vi "CleanUp.vi"(0 "object in":refnum<class "Hamamatsu.lvclass">, 5 "error in (no error)":errorcluster) -> (14 "object out":refnum<class "Hamamatsu.lvclass">, 19 "error out":errorcluster)   [LabVIEW 2021, in "Hamamatsu.lvclass"]
uses:
  Hamamatsu.lvclass
  Hamamatsu.lvclass/Hamamatsu.ctl
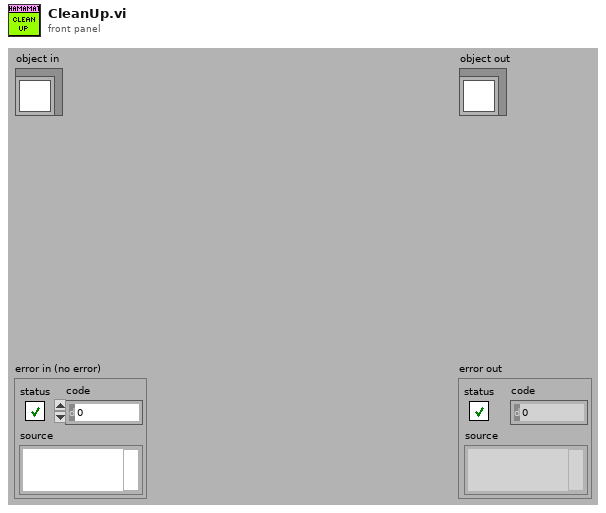
[diagram p1: front panel]
types:
  T1 = typedef "IMAQ Image.ctl" = refnum<image>
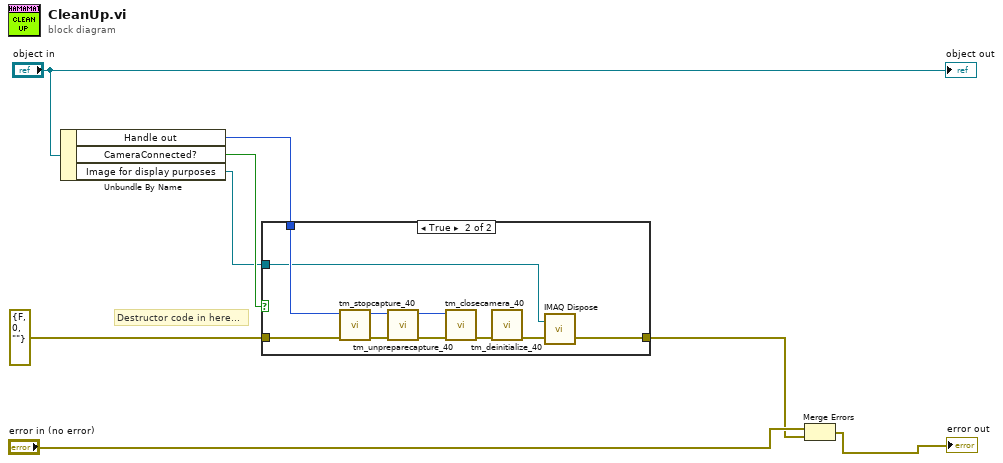
[diagram p0: block diagram]
diagram:
  # "Destructor code in here..."
  n1 = Unbundle By Name("object in") -> ("Handle out"=w5:u32, "CameraConnected?"=w2:bool, "Image for display purposes"=w1:T1)
  n2 = case shown="True" w2 {
    tunnel: w5 -> [_ w13]
    tunnel: errorcluster {"status"=FALSE, "code"=0, "source"=""} ("error in (no error)") -> [w9 w15]
    tunnel: [w9 w10] -> w3
    tunnel: w1 -> [_ w12]
    frame False {
    }
    frame True {
      n3 = call <userlib>:"tm_stopcapture_40.vi"("error in (no error)"=w15, "Handle in"=w13) -> ("error out"=w17:errorcluster, "Handle out"=w18:u32)  [unwired: 8 in]
      n4 = call <userlib>:"tm_unpreparecapture_40.vi"("error in (no error)"=w17, "Handle in"=w18) -> ("error out"=w16:errorcluster, "Handle out"=w14:u32)  [unwired: 8 in]
      n5 = call <userlib>:"tm_closecamera_40.vi"("error in (no error)"=w16, "Handle in"=w14) -> ("error out"=w19:errorcluster)  [unwired: 9 in]
      n6 = call <userlib>:"tm_deinitialize_40.vi"("error in (no error)"=w19) -> ("error out"=w11:errorcluster)  [unwired: 10 in]
      n7 = call "IMAQ Dispose"("Image"=w12, "error in (no error)"=w11) -> ("error out"=w10:errorcluster)  [unwired: 4 in]
    }
  }
  n8 = Merge Errors("error in (no error)", w3) -> (→"error out":errorcluster)
  "object out" <- "object in"
